vi "genSensorUpdatePacket.vi"(10 "node ID":u8) -> (3 "packet string":string)   [LabVIEW 2011]
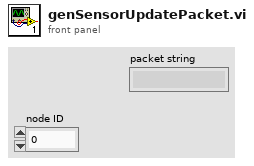
[diagram p1: front panel]
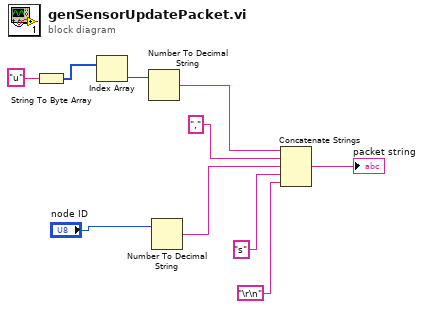
[diagram p0: block diagram]
diagram:
  n1 = String To Byte Array(string="u") -> (unsigned byte array=w9:u8[])
  n2 = Index Array(array=w9) -> (element=w8:u8)  [unwired: 1 in]
  n3 = Number To Decimal String(number=w8) -> (decimal integer string=w1:string)  [unwired: 1 in]
  n4 = Number To Decimal String(number="node ID") -> (decimal integer string=w6:string)  [unwired: 1 in]
  n5 = Concatenate Strings(w1, ",", w6, "s", "\r\n") -> (→"packet string":string)
